vi "ExampleTC01.vi"() -> ()   [LabVIEW 2012]
uses:
  <vilib>/DAQmx/read.llb/DAQmx Read.vi
  <vilib>/DAQmx/read.llb/DAQmx Read (Analog DBL 1Chan 1Samp).vi
  Instance           4 25Saved   LabVIEWTempLogger .vi
  <vilib>/DAQmx/miscellaneous.llb/DAQmx Fill In Error Info.vi
panel:
  in  "thermocouple type":i32(ring)=10072 items=["J"=10072, "K"=10073, "N"=10077, "R"=10082, "S"=10085, "T"=10086, "B"=10047, "E"=10055]
  out "data":dbl format="%0.2f"
  in  "Sampling Interval (s)":dbl=1.0 caption="Delay Time (s)"
  in  "Stop":bool
  # "NI USB-TC01 LabVIEW Temperature Logger"
  # "Switch to the block diagram (Window » Show Block Diagram) to configure the device, thermocouple type, and temperature unit."
  # "© 2010 National Instruments. All rights reserved."
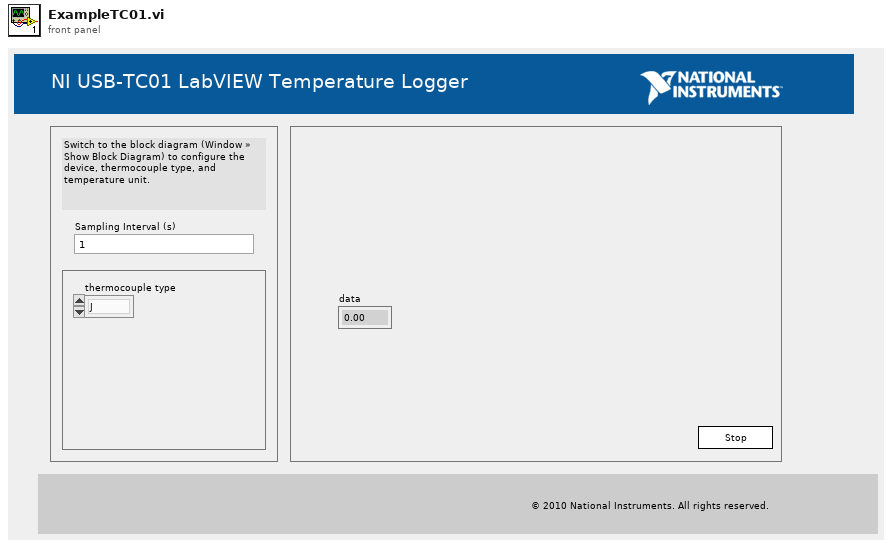
[diagram p1: front panel]
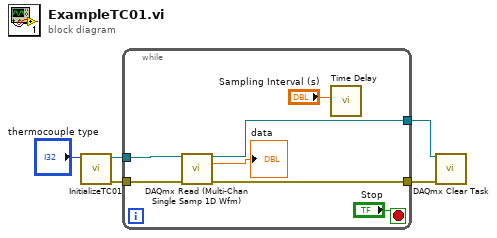
[diagram p0: block diagram]
diagram:
  n1 = call "InitializeTC01.vi"("thermocouple type"="thermocouple type") -> ("error out"=w2:errorcluster, "task out"=w3:refnum<k21>)  [unwired: 9 in]
  n2 = while {
    tunnel: [w9] -> w5
    tunnel: [w8] -> w4
    tunnel: w3 -> [w7]
    tunnel: w2 -> [w6]
    stop <- "Stop" stop-if-true
    n3 = call-poly "DAQmx Read (Multi-Chan Single Samp 1D Wfm).vi"("task/channels in"=w7, "error in"=w6) -> ("task out"=w9:refnum<k21>, "data"=→"data":dbl, "error out"=w8:errorcluster)  [unwired: 11 out]
    n4 = call "Time Delay"("Delay Time (s)"="Sampling Interval (s)") -> ()  [unwired: 10 in, 1 out]
  }
  n5 = call <vilib>:"DAQmx Clear Task.vi"("task in"=w5, "error in"=w4) -> ()  [unwired: 14 out]
